vi "FTS Get Instrument Property Model.vi"(8 "error in (no error)":errorcluster, 11 "specIndex":u16) -> (0 "error out":errorcluster, 3 "function return":u16)   [LabVIEW 2010, in "FTSLib.lvlib"]
doc: "INSTRUMENT_MODEL __cdecl FTS_GetInstrumentProperty_Model(unsigned short specIndex);"
uses:
  FTSLib.lvlib
  FTSLib.dll
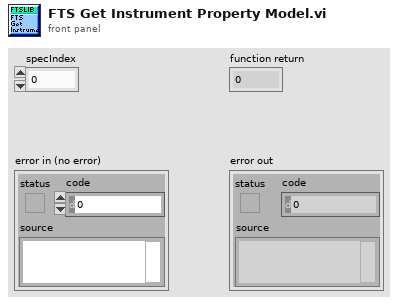
[diagram p1: front panel]
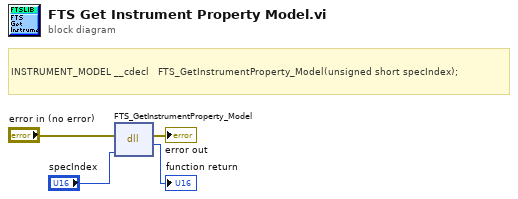
[diagram p0: block diagram]
diagram:
  # "INSTRUMENT_MODEL\t__cdecl   FTS_GetInstrumentProperty_Model(unsigned short specIndex);"
  n1 = dll-call lib="FTSLib.*" fn="FTS_GetInstrumentProperty_Model"(error in="error in (no error)", "specIndex"="specIndex") -> (error out=→"error out":errorcluster, →"function return":u16)  [unwired: 3 in, 1 out]
